vi "xxxxx.vi"(10 "String":string, 11 "jettl Msg xxxxx in":refnum<class "jettl Msg xxxxx.lvclass">) -> (3 "jettl Msg xxxxx out":refnum<class "jettl Msg xxxxx.lvclass">)   [LabVIEW 2021, in "jettl Tools.lvlib" / "jettl Msg xxxxx.lvlib" / "jettl Msg xxxxx.lvclass"]
uses:
  jettl Msg xxxxx.lvclass
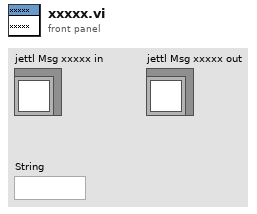
[diagram p1: front panel]
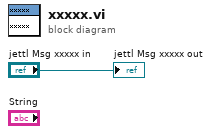
[diagram p0: block diagram]
diagram:
  "jettl Msg xxxxx out" <- "jettl Msg xxxxx in"
